vi "Create Client from Template.vi"(8 "error in (no error)":errorcluster, 9 "Generated Server Name":string="Generated Server", 10 "Target Project Path":path, 11 "Application ref in":refnum<vi>) -> (0 "error out":errorcluster, 3 "Server library out":refnum<vi>)   [LabVIEW 2019, in "gRPC Template Creation Utility.lvlib"]
uses:
  gRPC Template Creation Utility.lvlib
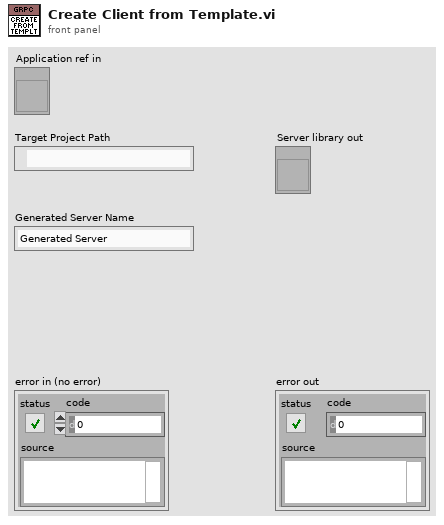
[diagram p1: front panel]
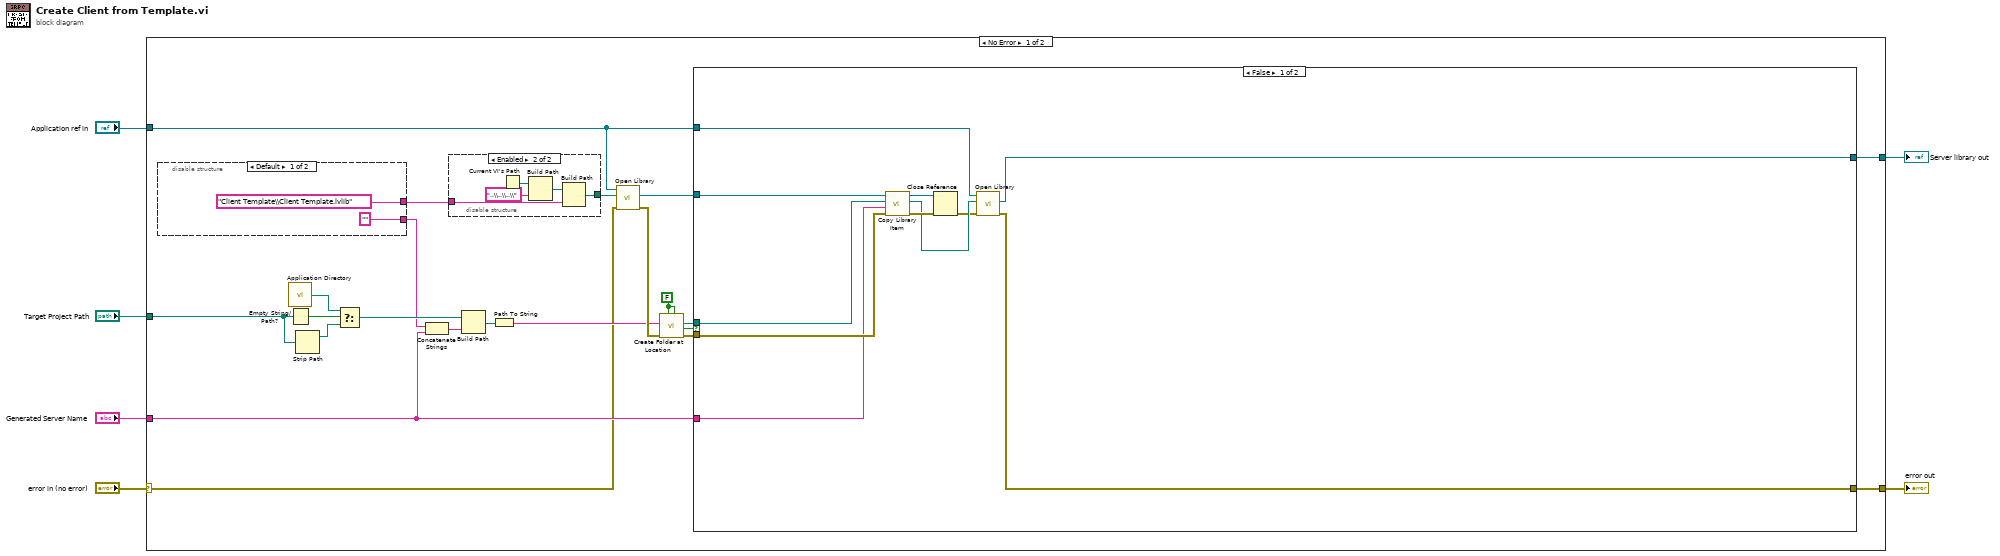
[diagram p0: block diagram]
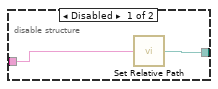
[diagram p2: hidden frame]
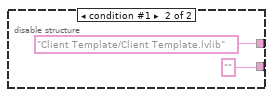
[diagram p3: hidden frame]
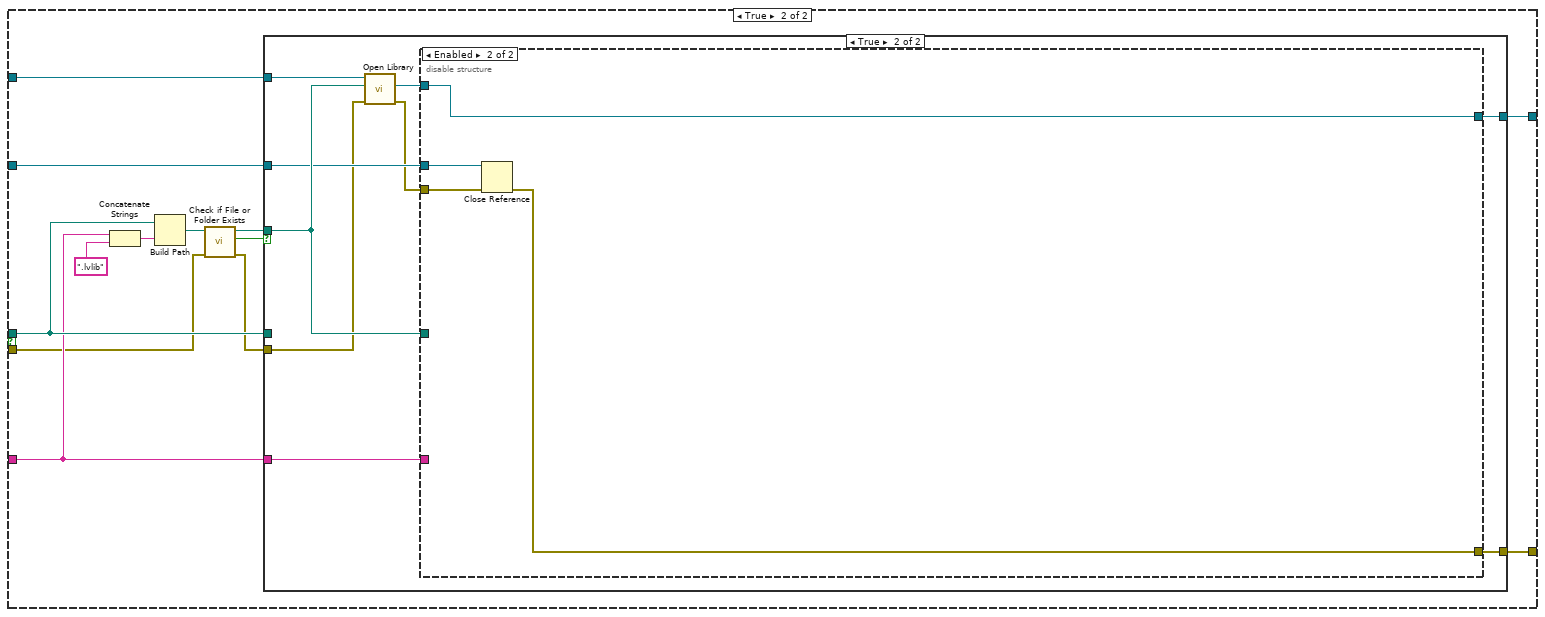
[diagram p4: hidden frame]
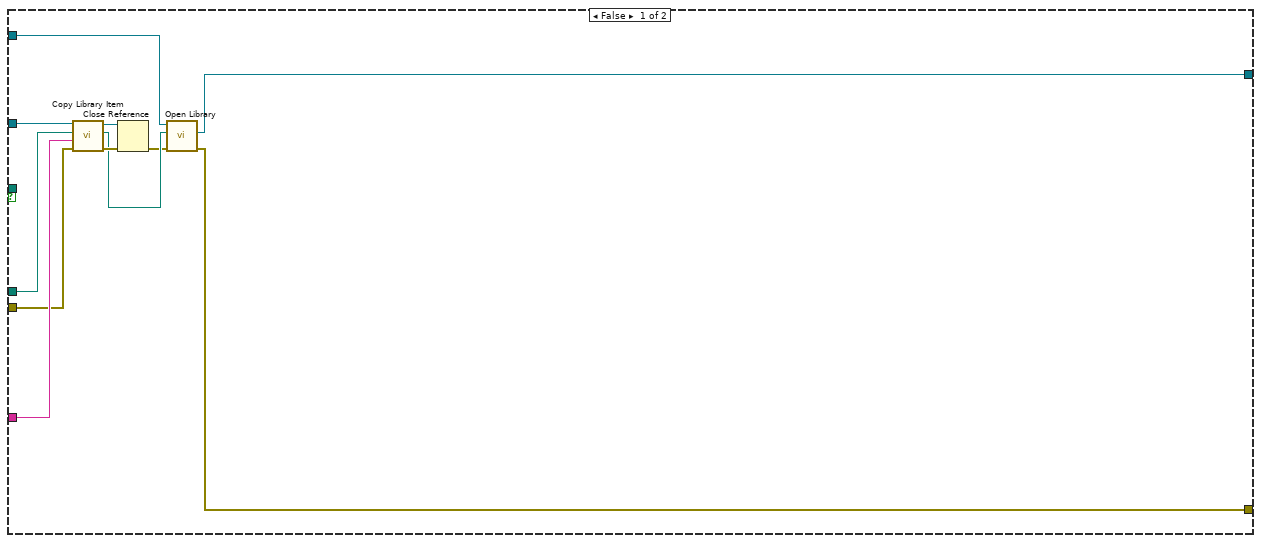
[diagram p5: hidden frame]
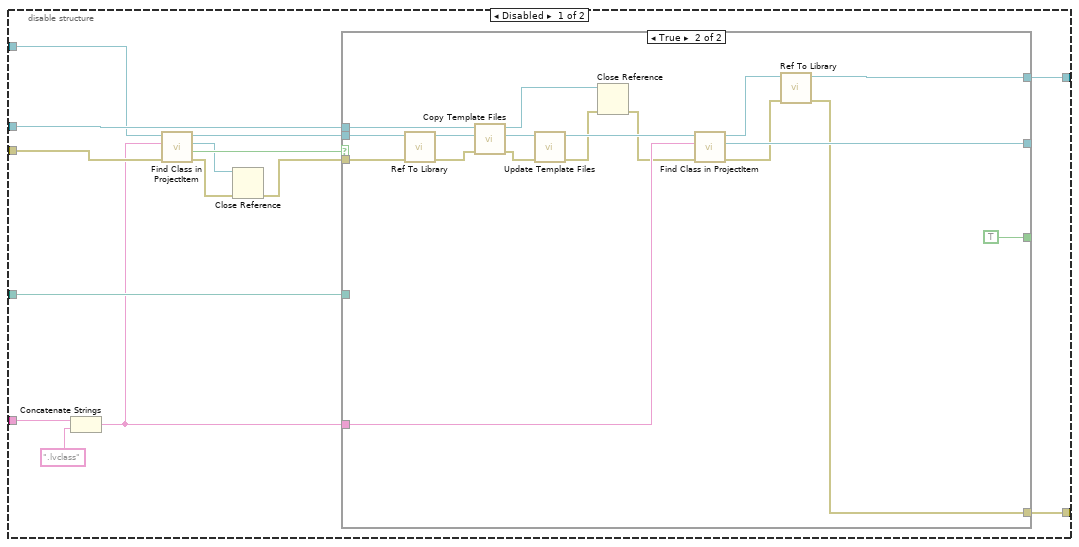
[diagram p6: hidden frame]
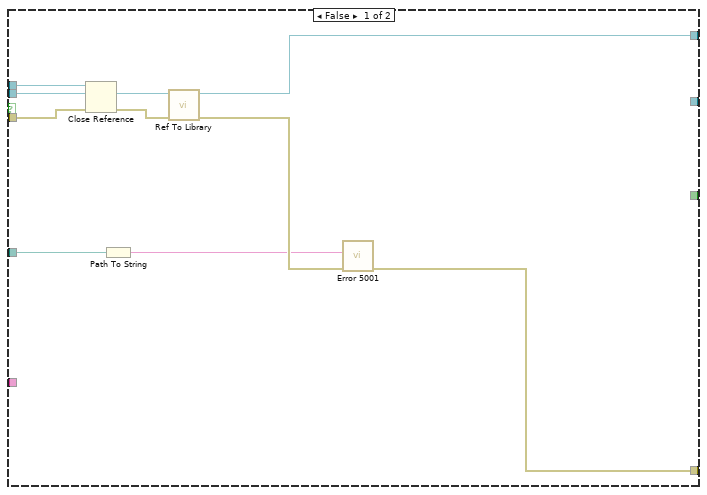
[diagram p7: hidden frame]
diagram:
  n1 = case shown="No Error" "error in (no error)" {
    selector: "error in (no error)" -> [w10 w129]
    tunnel: [w28 w129] -> w6
    tunnel: [w27 _] -> w5
    tunnel: "Target Project Path" -> [w13 _]
    tunnel: "Generated Server Name" -> [w12 _]
    tunnel: "Application ref in" -> [w11 _]
    frame No Error {
      w21 = FALSE ("Use Relative")
      n2 = disable-structure shown="Default" {
        disable-tunnel: ["Client Template\\Client Template.lvlib" ("Application Relative Path") "Client Template/Client Template.lvlib" ("Application Relative Path")] -> w8
        disable-tunnel: ["" ("Path") "" ("Path")] -> w7
        frame condition #0 (active) {
        }
        frame condition #1 {
        }
      }
      n3 = call <vilib>:"Application Directory.vi"() -> ("Application Directory"=w14:path)
      n4 = Empty String/Path?(string/path=w13) -> (empty?=w17:bool)
      n5 = Strip Path(path=w13) -> (stripped path=w16:path)  [unwired: 1 out]
      n6 = Select(t=w14, s=w17, f=w16) -> (s? t:f=w15:path)
      n7 = Concatenate Strings(w7, w12) -> (w20:string)
      n8 = disable-structure shown="Enabled" {
        disable-tunnel: [w30 w33] -> w24
        disable-tunnel: w8 -> [w29 w31]
        frame Disabled {
          n9 = call "Set Relative Path.vi"("Application Relative Path"=w29) -> ("Full Path"=w30:path)
        }
        frame Enabled {
          n10 = Current VI's Path() -> (path=w35:path)
          n11 = Build Path(base path=w35, name or relative path="..\\..\\..\\") -> (appended path=w32:path)
          n12 = Build Path(base path=w32, name or relative path=w31) -> (appended path=w33:path)
        }
      }
      n13 = Build Path(base path=w15, name or relative path=w20) -> (appended path=w19:path)
      n14 = Path To String(path=w19) -> (string=w18:string)
      n15 = call "Open Library.vi"("error in (no error)"=w10, "Full Path"=w24, "Application in"=w11) -> ("error out"=w25:errorcluster, "Library out"=w22:refnum<vi>)  [unwired: 6 in, 1 out]
      n16 = call "Create Folder at Location.vi"("Override existing (F)"=w21, "Use Relative (F)"=w21, "Error In"=w25, "Path"=w18) -> ("Error Out"=w26:errorcluster, "Already Exists ?"=w9:bool, "Full path out"=w23:path)  [unwired: 5 in]
      n17 = case shown="False" w9 {
        tunnel: [w42 w54] -> w28
        tunnel: [w50 w59] -> w27
        tunnel: w26 -> [w47 w52]
        tunnel: w23 -> [w46 w56]
        tunnel: w22 -> [w45 w57]
        tunnel: w12 -> [w41 w55]
        tunnel: w11 -> [w40 w58]
        frame False {
          n18 = call "Copy Library Item.vi"("error in (no error)"=w47, "Copy Name"=w41, "Copy location"=w46, "Library in"=w45) -> ("error out"=w49:errorcluster, "New Lib Path"=w44:path, "Library out"=w48:refnum<vi>)  [unwired: 5 in]
          n19 = Close Reference(reference=w48, error in (no error)=w49) -> (error out=w43:errorcluster)
          n20 = call "Open Library.vi"("error in (no error)"=w43, "Full Path"=w44, "Application in"=w40) -> ("error out"=w42:errorcluster, "Library out"=w50:refnum<vi>)  [unwired: 6 in, 1 out]
        }
        frame True {
          n21 = Concatenate Strings(w55, ".lvlib" ("string")) -> (w62:string)
          n22 = Build Path(base path=w56, name or relative path=w62) -> (appended path=w61:path)
          n23 = call <vilib>:"Check if File or Folder Exists.vi"("error in (no error)"=w52, "path"=w61) -> ("error out"=w51:errorcluster, "file or folder exists?"=w60:bool, "dup path"=w53:path)  [unwired: 7 in]
          n24 = case shown="True" w60 {
            tunnel: [w69 w81] -> w59
            tunnel: w58 -> [w68 w83]
            tunnel: w57 -> [w67 w78]
            tunnel: w56 -> [w66 _]
            tunnel: w55 -> [w65 w82]
            tunnel: w51 -> [w64 w77]
            tunnel: [w70 w80] -> w54
            tunnel: w53 -> [_ w79]
            frame False {
              n25 = call "Copy Library Item.vi"("error in (no error)"=w64, "Copy Name"=w65, "Copy location"=w66, "Library in"=w67) -> ("error out"=w74:errorcluster, "New Lib Path"=w72:path, "Library out"=w73:refnum<vi>)  [unwired: 5 in]
              n26 = Close Reference(reference=w73, error in (no error)=w74) -> (error out=w71:errorcluster)
              n27 = call "Open Library.vi"("error in (no error)"=w71, "Full Path"=w72, "Application in"=w68) -> ("error out"=w70:errorcluster, "Library out"=w69:refnum<vi>)  [unwired: 6 in, 1 out]
            }
            frame True {
              n28 = call "Open Library.vi"("error in (no error)"=w77, "Full Path"=w79, "Application in"=w83) -> ("error out"=w75:errorcluster, "Library out"=w76:refnum<vi>)  [unwired: 6 in, 1 out]
              n29 = disable-structure shown="Enabled" {
                disable-tunnel: w82 -> [w97 _]
                disable-tunnel: [w96 w128] -> w81
                disable-tunnel: [w95 w125] -> w80
                disable-tunnel: w79 -> [w94 _]
                disable-tunnel: w78 -> [w93 w127]
                disable-tunnel: w76 -> [w92 w128]
                disable-tunnel: w75 -> [w90 w126]
                frame Disabled {
                  n30 = Concatenate Strings(w97, ".lvclass" ("Class Name")) -> (w84:string)
                  n31 = call "Find Class in ProjectItem.vi"("error in (no error)"=w90, "Class Name"=w84, "ProjectItem in"=w92) -> ("error out"=w86:errorcluster, "Found?"=w88:bool, "LVClass out"=w87:refnum<vi>, "ProjectItem out"=w89:refnum<vi>)  [unwired: 5 in]
                  n32 = Close Reference(reference=w87, error in (no error)=w86) -> (error out=w85:errorcluster)
                  n33 = case shown="True" w88 {
                    tunnel: w89 -> [w106 w119]
                    tunnel: [w105 w124] -> w96
                    tunnel: w85 -> [w100 w121]
                    tunnel: [w103 w112] -> w95
                    tunnel: w94 -> [w102 _]
                    tunnel: [_ TRUE] -> _
                    tunnel: w93 -> [w101 w111]
                    tunnel: w84 -> [_ w118]
                    tunnel: [_ w117] -> _
                    frame False {
                      n34 = Close Reference(reference=w101, error in (no error)=w100) -> (error out=w99:errorcluster)
                      n35 = Path To String(path=w102) -> (string=w98:string)
                      n36 = call "Ref To Library.vi"("error in (no error)"=w99, "ProjectItem in"=w106) -> ("error out"=w104:errorcluster, "Library out"=w105:refnum<vi>)  [unwired: 8 in]
                      n37 = call "Error 5001.vi"("error in (no error)"=w104, "Server Class Path"=w98) -> ("error out"=w103:errorcluster)  [unwired: 9 in]
                    }
                    frame True {
                      n38 = call "Ref To Library.vi"("error in (no error)"=w121, "ProjectItem in"=w119) -> ("error out"=w120:errorcluster, "Library out"=w122:refnum<vi>)  [unwired: 8 in]
                      n39 = call "Copy Template Files.vi"("error in (no error)"=w120, "Server Library (Library Item) in"=w122, "Template Library (Library Item) in"=w111) -> ("error out"=w110:errorcluster, "Server Library (Library Item) out"=w109:refnum<vi>, "Template Library (Library Item) out"=w107:refnum<vi>)  [unwired: 6 in]
                      n40 = call "Update Template Files.vi"("error in (no error)"=w110, "Server Library (Library Item) in"=w109) -> ("error out"=w108:errorcluster, "Server Library (Library Item) out"=w116:refnum<vi>)  [unwired: 8 in]
                      n41 = Close Reference(reference=w107, error in (no error)=w108) -> (error out=w114:errorcluster)
                      n42 = call "Find Class in ProjectItem.vi"("error in (no error)"=w114, "Class Name"=w118, "ProjectItem in"=w116) -> ("error out"=w113:errorcluster, "LVClass out"=w117:refnum<vi>, "ProjectItem out"=w115:refnum<vi>)  [unwired: 5 in, 1 out]
                      n43 = call "Ref To Library.vi"("error in (no error)"=w113, "ProjectItem in"=w115) -> ("error out"=w112:errorcluster, "Library out"=w124:refnum<vi>)  [unwired: 8 in]
                    }
                  }
                }
                frame Enabled {
                  n44 = Close Reference(reference=w127, error in (no error)=w126) -> (error out=w125:errorcluster)
                }
              }
            }
          }
        }
      }
    }
    frame Error {
    }
  }
  "error out" <- w6
  "Server library out" <- w5
